vi "Rev 1.vi"() -> ()   [LabVIEW 2018]
uses:
  5e9b011a-7452-4143-b5bd-a1605937e046.vi
  7c459f28-9012-48fc-b39f-7befdbae034b.vi
  <vilib>/Analysis/baseanly.llb/Mean (DBL).vi
  <vilib>/Analysis/NI_AALBase.lvlib
panel:
  in  "?":bool
  in  "?":T1(tab)
  in  "Refresh Data":bool
  out "?":string
  out "?":string
  in  "Time Scale (hours)":u32(slide) scale=0.0..168.0
  in  "?":enum32{"Graph"}(tab)
  out "Temp v Time":cluster{"all rows":dbl[], "all rows":dbl[]}(graph)
  out "Minimum Temperature":dbl
  out "Maximum Temperature":dbl
  out "Thermometer":dbl(slide) scale=0.0..100.0
  out "Mean Temp":dbl
  in  "?":enum32{"Graph"}(tab)
  out "Humidity v time":cluster{dbl[], dbl[]}(graph)
  out "Minimum Humidity":dbl
  out "Maximum Humidity":dbl
  out "Hygrometer":dbl(slide) scale=0.0..100.0
  out "Average Humidity":dbl
  out "Minimum Luminance":dbl
  out "Maximum Luminance":dbl
  in  "?":enum32{"Graph"}(tab)
  out "Luminance v time":cluster{dbl[], dbl[]}(graph)
  out "Luminance":dbl(knob) scale=6.0..6000.0
  out "Average Luminance":dbl
  # "°F"
  # "°F"
  # "°F"
  # "Oldest"
  # "Most Recent"
  # "%"
  # "%"
  # "%"
  # "Oldest"
  # "Most Recent"
  # "Lumens"
  # "Lumens"
  # "Lumens"
  # "Oldest"
  # "Most Recent"
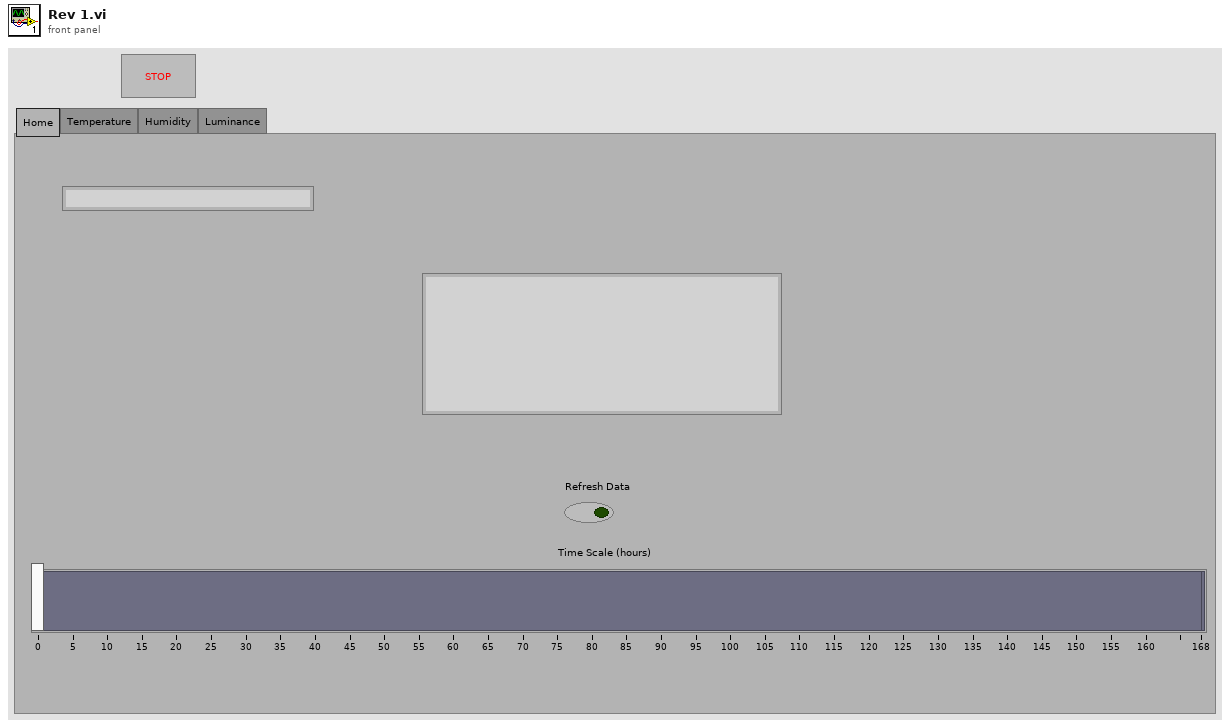
[diagram p1: front panel]
types:
  T1 = enum32{"Home", "Temperature", "Humidity", "Luminance"}
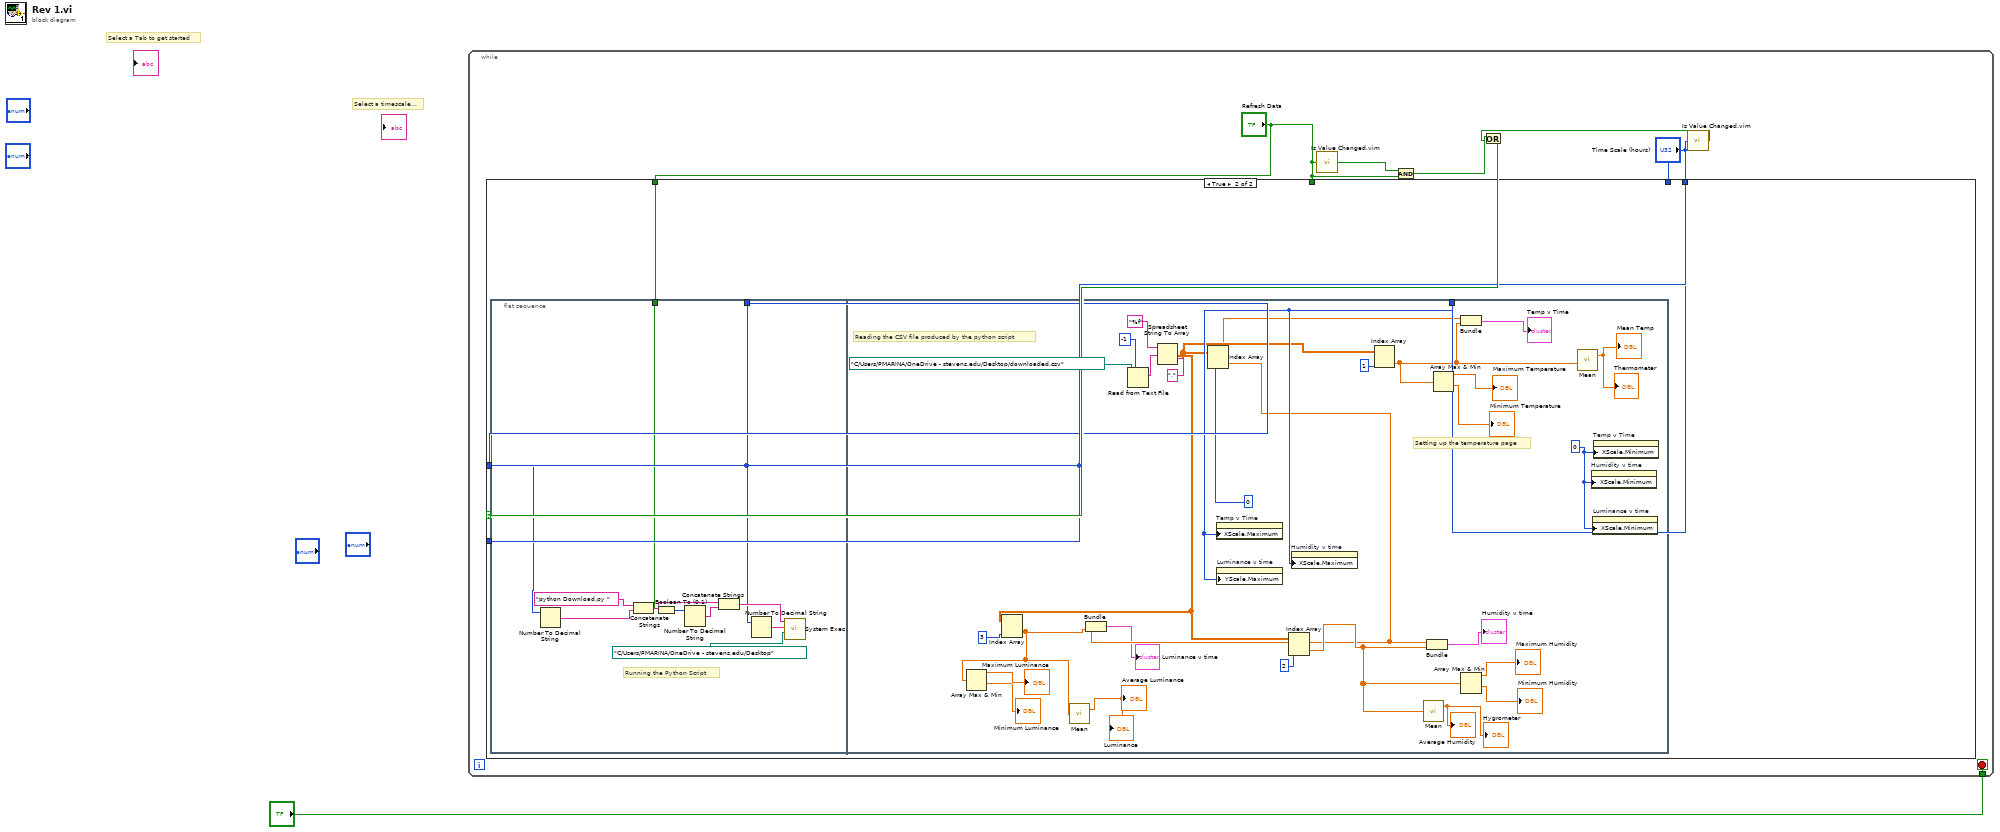
[diagram p0: block diagram]
diagram:
  # "Select a timescale..."
  # "Select a Tab to get started"
  n1 = while {
    tunnel: "?" -> [w8]
    stop <- w8 stop-if-true
    n2 = call "Is Value Changed.vim"("value"="Refresh Data") -> ("changed or first call?"=w7:bool)
    n3 = And(x=w7, y="Refresh Data") -> (x .and. y?=w6:bool)
    n4 = call "Is Value Changed.vim"("value"="Time Scale (hours)") -> ("changed or first call?"=w5:bool)
    n5 = Or(x=w6, y=w5) -> (x .or. y?=w4:bool)
    n6 = case shown="True" w4 {
      tunnel: "Time Scale (hours)" -> [_ _]
      tunnel: "Time Scale (hours)" -> [_ w11]
      tunnel: "Refresh Data" -> [_ _]
      tunnel: "Time Scale (hours)" -> [_ w10]
      tunnel: "Time Scale (hours)" -> [_ _]
      tunnel: "Refresh Data" -> [_ w9]
      frame False {
      }
      frame True {
        n7 = flat-sequence {
          tunnel: w9 -> [w13]
          tunnel: w11 -> [w12]
          tunnel: w10 -> [w33]
          frame #0 {
            # "Running the Python Script"
            n8 = Number To Decimal String(number=w12) -> (decimal integer string=w18:string)  [unwired: 1 in]
            n9 = Concatenate Strings("python Download.py ", w18) -> (w14:string)
            n10 = Boolean To (0,1)(Boolean=w13) -> (0, 1=w17:i16)
            n11 = Number To Decimal String(number=w17) -> (decimal integer string=w16:string)  [unwired: 1 in]
            n12 = Concatenate Strings(w14, w16) -> (w15:string)
            n13 = Number To Decimal String(number=w12) -> (decimal integer string=w19:string)  [unwired: 1 in]
            n14 = call <vilib>:"System Exec.vi"("working directory"=path "C:/Users/PMARINA/OneDrive - stevens.edu/Desktop", "standard input"=w19, "command line"=w15) -> ()  [unwired: 5 in, 4 out]
          }
          frame #1 {
            w32 = 0
            # "Setting up the temperature page"
            # "Reading the CSV file produced by the python script"
            n15 = Read from Text File(file (use dialog)=path "C:/Users/PMARINA/OneDrive - stevens.edu/Desktop/downloaded.csv", count=-1) -> (text=w43:string)  [unwired: 2 in, 3 out]
            n16 = Spreadsheet String To Array(delimiter (Tab)=",", format string="%f", spreadsheet string=w43) -> (array=w27:dbl[][])  [unwired: 1 in]
            n17 = Index Array(array=w27, index (col)=3) -> (element=w25:dbl[])  [unwired: 1 in]
            n18 = Array Max & Min(array=w25) -> (max value=→"Maximum Luminance":dbl, min value=→"Minimum Luminance":dbl)  [unwired: 2 out]
            n19 = call-poly <vilib>:"Mean.vi"("X"=w25) -> ("mean"=→"Average Luminance" →"Luminance":dbl)  [unwired: 1 out]
            n20 = Index Array(array=w27, index (col)=0) -> (element=w24:dbl[])  [unwired: 1 in]
            n21 = Bundle(w24, w25) -> (→"Luminance v time":cluster{dbl[], dbl[]})  [unwired: 1 in]
            n22 = property on="Temp v Time" class="XYGraph (strict)"("XScale.Maximum"=w33) -> ()  [unwired: 2 in, 2 out]
            n23 = property on="Luminance v time" class="XYGraph (strict)"("YScale.Maximum"=w33) -> ()  [unwired: 2 in, 2 out]
            n24 = Index Array(array=w27, index (col)=2) -> (element=w26:dbl[])  [unwired: 1 in]
            n25 = property on="Humidity v time" class="XYGraph (strict)"("XScale.Maximum"=w33) -> ()  [unwired: 2 in, 2 out]
            n26 = Index Array(array=w27, index (col)=1) -> (element=w30:dbl[])  [unwired: 1 in]
            n27 = call-poly <vilib>:"Mean.vi"("X"=w26) -> ("mean"=→"Hygrometer" →"Average Humidity":dbl)  [unwired: 1 out]
            n28 = Bundle(w24, w26) -> (→"Humidity v time":cluster{dbl[], dbl[]})  [unwired: 1 in]
            n29 = Array Max & Min(array=w30) -> (max value=→"Maximum Temperature":dbl, min value=→"Minimum Temperature":dbl)  [unwired: 2 out]
            n30 = Bundle(w24, w30) -> (→"Temp v Time":cluster{dbl[], dbl[]})  [unwired: 1 in]
            n31 = Array Max & Min(array=w26) -> (max value=→"Maximum Humidity":dbl, min value=→"Minimum Humidity":dbl)  [unwired: 2 out]
            n32 = call-poly <vilib>:"Mean.vi"("X"=w30) -> ("mean"=→"Thermometer" →"Mean Temp":dbl)  [unwired: 1 out]
            n33 = property on="Humidity v time" class="XYGraph (strict)"("XScale.Minimum"=w32) -> ()  [unwired: 2 in, 2 out]
            n34 = property on="Luminance v time" class="XYGraph (strict)"("XScale.Minimum"=w32) -> ()  [unwired: 2 in, 2 out]
            n35 = property on="Temp v Time" class="XYGraph (strict)"("XScale.Minimum"=w32) -> ()  [unwired: 2 in, 2 out]
          }
        }
      }
    }
  }
